vi "PJ1_GG - Copy1.vi"() -> ()   [LabVIEW 2024]
uses:
  contol_vr 23/Control 9.ctl
  <vilib>/Instr/_visa.llb/VISA Configure Serial Port (Instr).vi
  <vilib>/express/express analysis/Spectral/Block/exnSpectralBlock spectral measurements PSD poly.vi
  <vilib>/express/express analysis/Spectral/Block/exnSpectralBlock spectral measurements PSD DDT.vi
  <vilib>/express/express analysis/Spectral/XNode/ExpressSpectralMeasurementsBlockNode.xnode
panel:
  out "Array":dbl[](array[numeric])
  out "appended array 2":dbl[](array[numeric])
  out "element":dbl
  out "data out":string
  in  "Sample":i32
  in  "Rate":dbl
  in  "Upper Cut-Off":dbl=40.0
  out "PSD":dynamicdata(graph)
  out "PSD MAX":dbl
  out "Index ที่มากที่สุด":i32
  out "max value":dbl
  out "B 18+1":dbl
  out "N 18+1":dbl
  in  "Aj 18+1":dbl
  out "B 18+1":dbl
  out "PSD 18+1":dbl
  out "B 18":dbl
  out "N 18":dbl
  in  "Aj 18":dbl
  out "B 18":dbl
  out "PSD 18":dbl
  out "B 18-1":dbl
  out "N 18-1":dbl
  in  "Aj 18-1":dbl
  out "B 18-1":dbl
  out "PSD 18-1":dbl
  out "9 Hz":dbl[](array[numeric])
  out "Max Index 9":i32
  out "PSD max 9":dbl
  out "PSD 9-1":dbl
  out "B 9-1":dbl
  in  "Aj 9-1":dbl
  out "N 9-1":dbl
  out "B 9-1":dbl
  out "PSD 9":dbl
  out "B 9":dbl
  in  "Aj 9":dbl
  out "N 9":dbl
  out "B 9":dbl
  out "PSD 9+1":dbl
  out "B 9+1":dbl
  in  "Aj 9+1":dbl
  out "N 9+1":dbl
  out "B 9+1":dbl
  out "8 Hz":dbl[](array[numeric])
  out "Max Index 8":i32
  out "PSD max 8":dbl
  out "B 16+1":dbl
  out "N 16+1":dbl
  in  "Aj  16+1":dbl
  out "B 16+1":dbl
  out "PSD  16+1":dbl
  out "B 16":dbl
  out "N  16":dbl
  in  "Aj  16":dbl
  out "B 16":dbl
  out "PSD  16":dbl
  out "B 16-1":dbl
  out "N  16-1":dbl
  in  "Aj   16-1":dbl
  out "B   16-1":dbl
  out "PSD 16-1":dbl
  out "B 8+1":dbl
  out "N 8+1":dbl
  in  "Aj  8+1":dbl
  out "B  8+1":dbl
  out "PSD 8+1":dbl
  out "B 8":dbl
  out "N  8":dbl
  in  "Aj  8":dbl
  out "B  8":dbl
  out "PSD 8":dbl
  out "B 8-1":dbl
  out "N  8-1":dbl
  in  "Aj  8-1":dbl
  out "B  8-1":dbl
  out "PSD 8-1":dbl
  out "PSD 14+1":dbl
  out "B 14+1":dbl
  in  "Aj 14+1":dbl
  out "N 14+1":dbl
  out "B 14+1":dbl
  out "PSD 14":dbl
  out "B 14":dbl
  in  "Aj 14":dbl
  out "N 14":dbl
  out "B 14":dbl
  out "PSD 14-1":dbl
  out "B 14-1":dbl
  in  "Aj 14-1":dbl
  out "N 14-1":dbl
  out "B 14-1":dbl
  out "PSD7+1":dbl
  out "B7+1":dbl
  in  "Aj7+1":dbl
  out "N7+1":dbl
  out "B7+1":dbl
  out "PSD 7":dbl
  out "B 7":dbl
  in  "Aj 7":dbl
  out "N7":dbl
  out "B7":dbl
  out "7 Hz":dbl[](array[numeric])
  out "Max Index 7":i32
  out "PSD max 7":dbl
  out "PSD 7-1":dbl
  out "B 7-1":dbl
  in  "Aj 7-1":dbl
  out "N7-1":dbl
  out "B7-1":dbl
  out "B12-1":dbl
  out "N12-1":dbl
  in  "Aj 12-1":dbl
  out "B 12-1":dbl
  out "PSD 12-1":dbl
  out "B12":dbl
  out "N12":dbl
  in  "Aj 12":dbl
  out "B12":dbl
  out "PSD 12":dbl
  out "B12+1":dbl
  out "N12+1":dbl
  in  "Aj 12+1":dbl
  out "B 12+1":dbl
  out "PSD 12+1":dbl
  out "B6+1":dbl
  out "N6+1":dbl
  in  "Aj 6+1":dbl
  out "B 6+1":dbl
  out "PSD 6+1":dbl
  out "B6":dbl
  out "N6":dbl
  in  "Aj 6":dbl
  out "B6":dbl
  out "PSD 6":dbl
  out "PSD 6-1":dbl
  out "6 Hz":dbl[](array[numeric])
  out "Max Index 6":i32
  out "PSD max 6":dbl
  out "B 6-1":dbl
  in  "Aj 6-1":dbl
  out "N6-1":dbl
  out "B6-1":dbl
  in  "Baseline":bool
  out "appended array":dbl[][](array[numeric])
  out "Filtered Signal":dynamicdata(graph)
  in  "Lower Cut-Off":dbl=1.0
  out "?":bool
  out "?":bool
  out "?":bool
  out "?":bool
  out "?":bool
  out "?":bool
  out "?":bool
  out "?":bool
  out "?":bool
  out "?":bool
  out "?":bool=TRUE
  out "?":bool=TRUE
  out "?":bool=TRUE
  out "?":bool=TRUE
  out "?":bool=TRUE
  out "?":bool=TRUE
  out "?":bool=TRUE
  out "?":bool=TRUE
  out "?":bool=TRUE
  out "?":bool=TRUE
  out "?":bool
  out "?":bool
  out "?":bool
  out "?":bool
  out "?":bool
  out "?":bool
  out "?":bool
  out "?":bool
  out "?":bool
  out "?":bool
  out "?":bool=TRUE
  out "?":bool=TRUE
  out "?":bool=TRUE
  out "?":bool=TRUE
  out "?":bool=TRUE
  out "?":bool=TRUE
  out "?":bool=TRUE
  out "?":bool=TRUE
  out "?":bool=TRUE
  out "?":bool=TRUE
  out "?":bool
  out "?":bool
  out "?":bool
  out "?":bool
  out "?":bool
  out "?":bool
  out "?":bool
  out "?":bool
  out "?":bool
  out "?":bool
  out "?":bool=TRUE
  out "?":bool=TRUE
  out "?":bool=TRUE
  out "?":bool=TRUE
  out "?":bool=TRUE
  out "?":bool=TRUE
  out "?":bool=TRUE
  out "?":bool=TRUE
  out "?":bool=TRUE
  out "?":bool=TRUE
  out "?":bool
  out "?":bool
  out "?":bool
  out "?":bool
  out "?":bool
  out "?":bool
  out "?":bool
  out "?":bool
  out "?":bool
  out "?":bool
  out "?":bool=TRUE
  out "?":bool=TRUE
  out "?":bool=TRUE
  out "?":bool=TRUE
  out "?":bool=TRUE
  out "?":bool=TRUE
  out "?":bool=TRUE
  out "?":bool=TRUE
  out "?":bool=TRUE
  out "?":bool=TRUE
  out "9 HZ":bool
  out "8 HZ":bool
  out "6 HZ":bool
  out "7 HZ":bool
  in  "Tab Control":enum32{"TAB 1", "TAB 2", "TAB 3", "TAB 4"}(tab)
  out "555":bool
  in  "MENU 4":bool
  in  "MENU 3":bool
  in  "MENU 2":bool
  in  "MENU":bool
  in  "start":bool
  in  "Text3":bool
  in  "Text2":bool
  in  "Backpage 2":T1
  out "String":string
  in  "Text1":bool
  in  "send":bool
  in  "Back":bool
  in  "1 3":bool
  in  "1 2":bool
  in  "1":bool
  out "String 2":string
  in  "SOS CALLING":bool
  in  "Blank Button 14":bool
  in  "LED":bool
  in  "Blank Button 12":bool
  in  "Back 4":bool
  in  "VISA resource name":refnum<visa-resource-name>
  # "Tel."
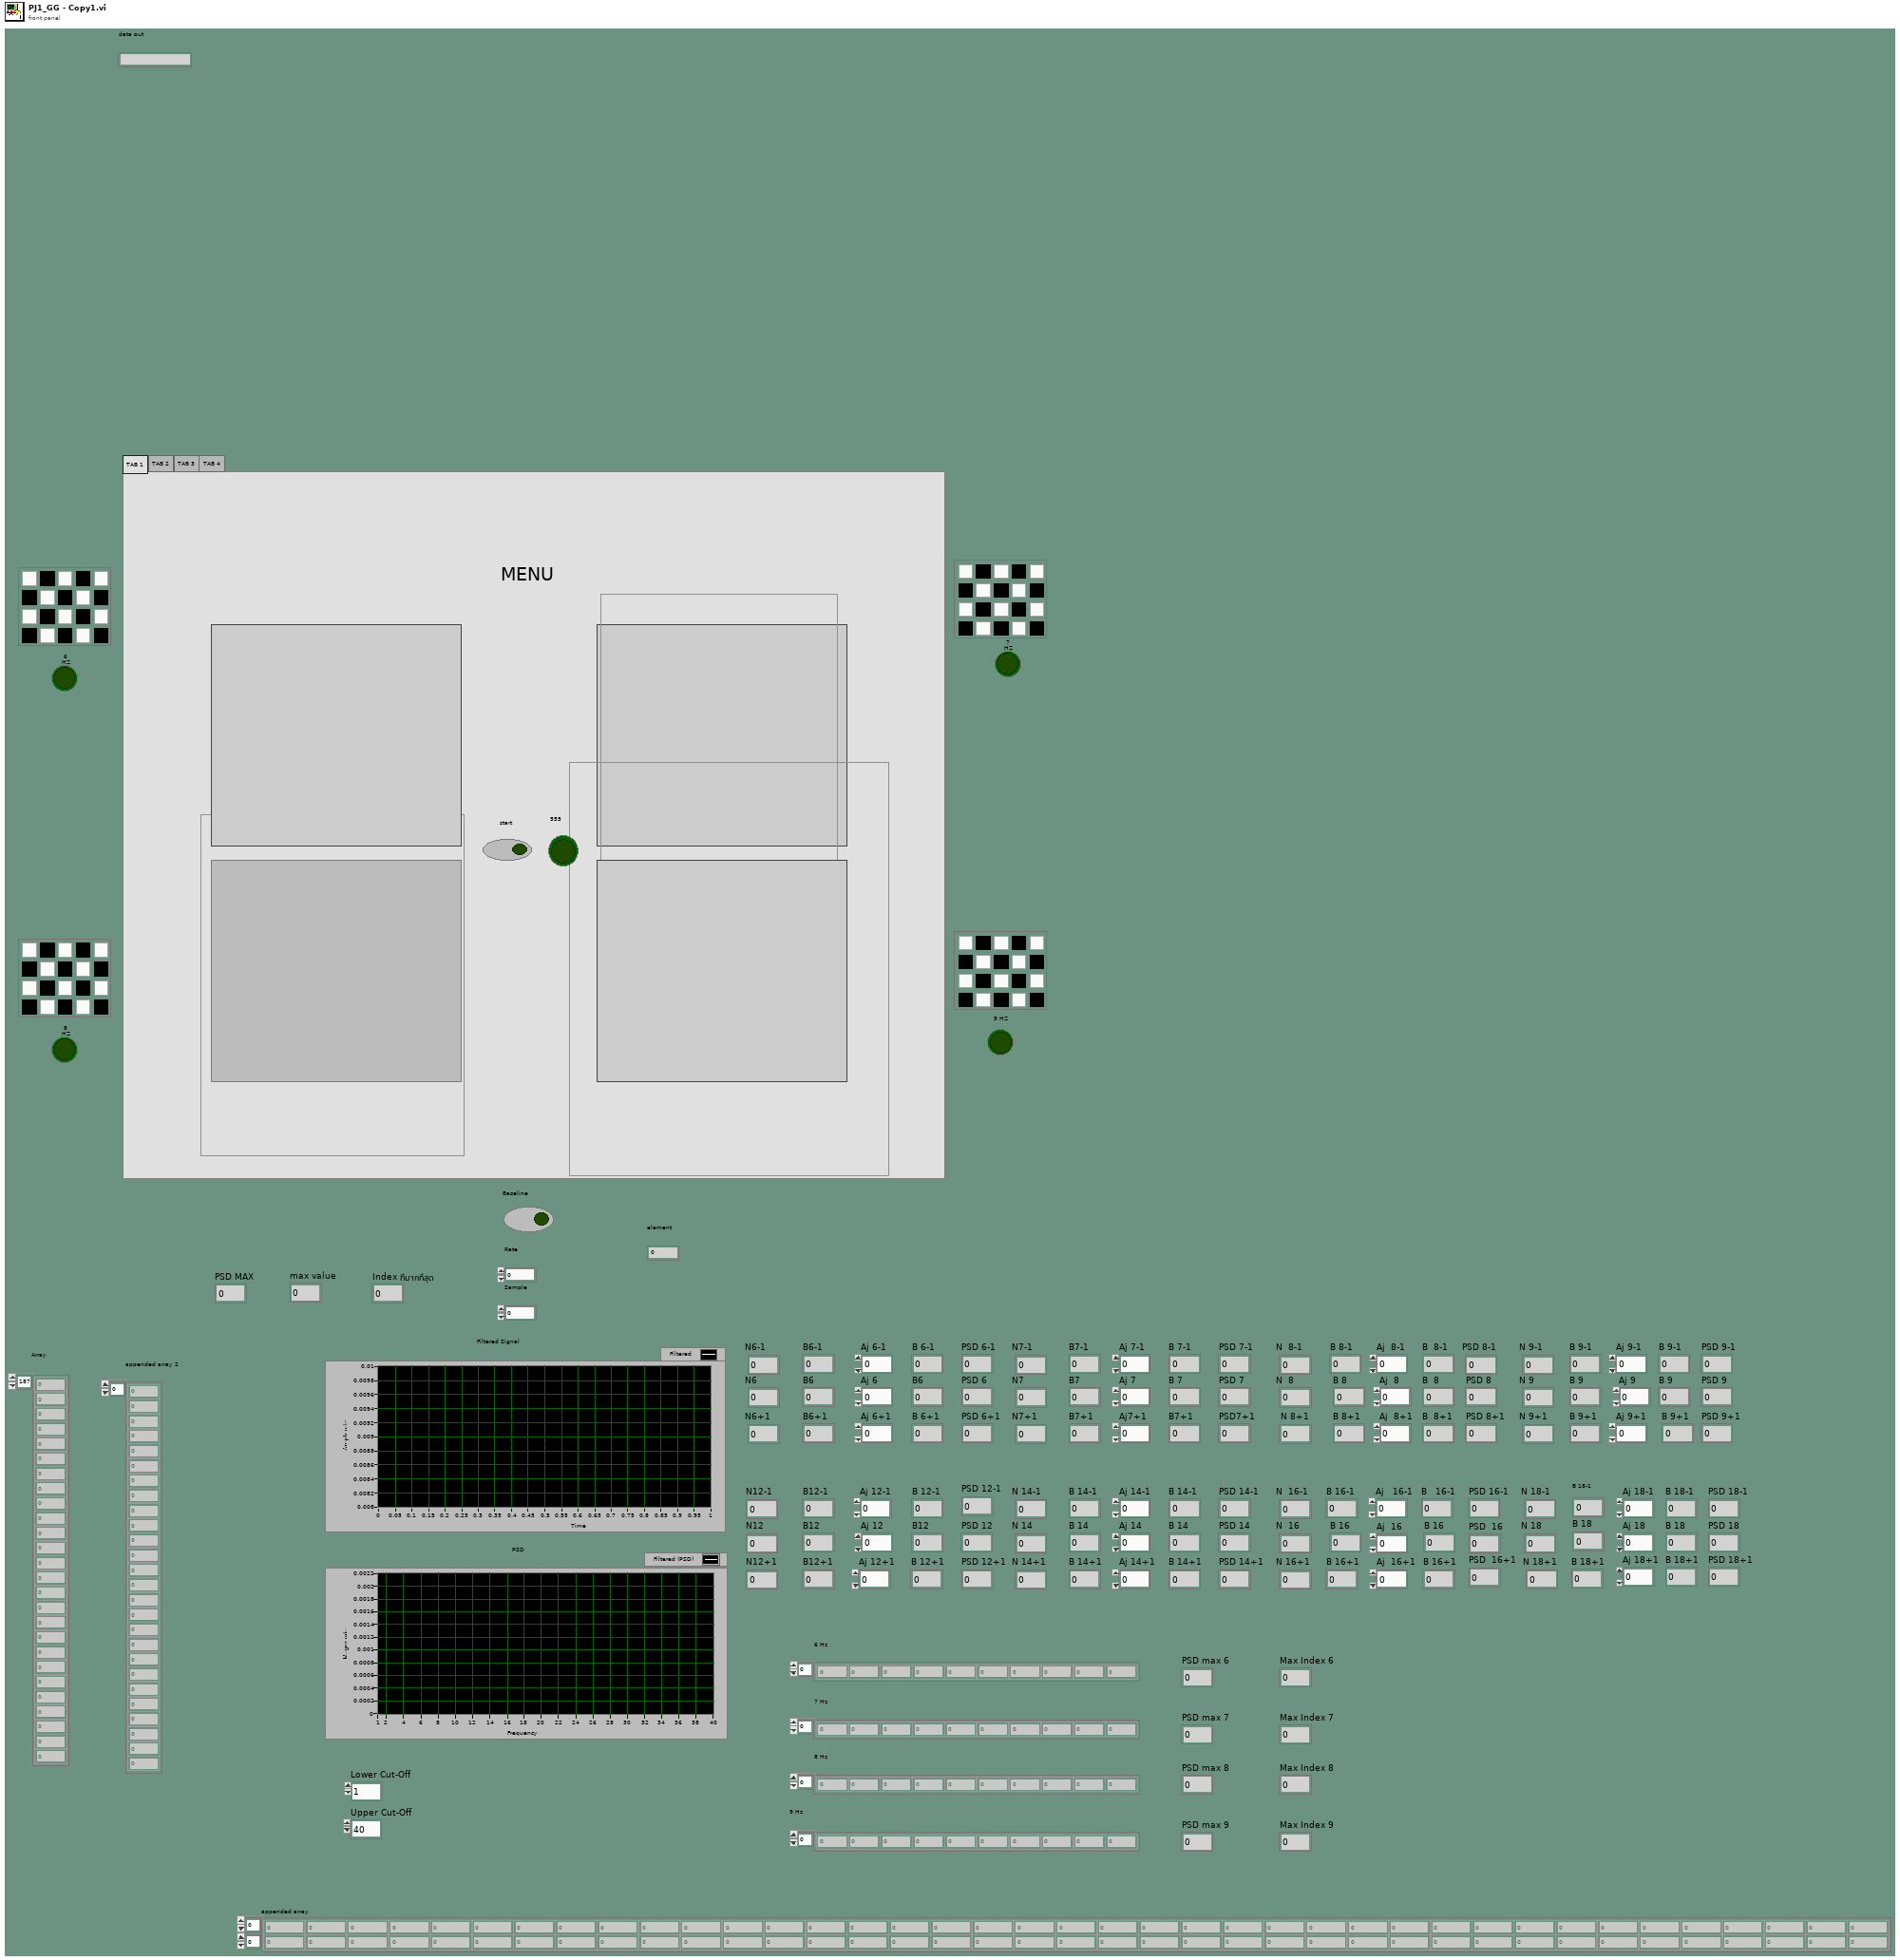
[diagram p1: front panel]
types:
  T1 = typedef "Control 9.ctl" = bool
  T2 = cluster{"averaging mode":u16, "weighting mode":u16, "number of averages":u32}
  T3 = cluster{"dB On (F)":bool, "unwrap phase (F)":bool, "convert to degree (F)":bool}
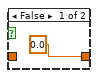
[diagram p3: hidden frame]
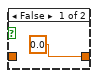
[diagram p5: hidden frame]
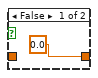
[diagram p7: hidden frame]
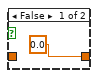
[diagram p9: hidden frame]
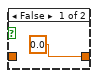
[diagram p11: hidden frame]
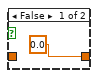
[diagram p13: hidden frame]
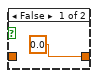
[diagram p15: hidden frame]
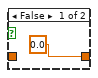
[diagram p17: hidden frame]
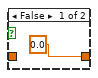
[diagram p19: hidden frame]
diagram:
  n1 = while {
    tunnel: [w15] -> _
    tunnel: [w16] -> _
    stop <- FALSE stop-if-true
    n2 = Obtain Queue(name (unnamed)="buffer", element data type=0.0) -> (queue out=w10:refnum<queue>, error out=w9:errorcluster)  [unwired: 3 in, 1 out]
    n3 = Obtain Queue(name (unnamed)="ganglion", element data type=0.0) -> (queue out=w16:refnum<queue>, error out=w15:errorcluster)  [unwired: 3 in, 1 out]
    n4 = while {
      tunnel: w16 -> [w535]
      tunnel: w15 -> [w534]
      shift-right: [w524] -> _
      shift-left: _ -> [_]
      tunnel: w10 -> [w531]
      tunnel: w9 -> [w530]
      tunnel: [w529] -> w12
      tunnel: [w528] -> w11
      stop <- FALSE stop-if-true
      # "เงื่อนไข while"
      n5 = for {
        N: 200 -> [_]
        shift-right: [w537] -> w524
        shift-left: dbl[] [] -> [w539]
        tunnel: [w544] -> _
        tunnel: w534 -> [w545]
        tunnel: [w541] -> _
        tunnel: [w540] -> _
        tunnel: w535 -> [w544]
        # "เคลีย 800 ก่อน"
        # "ตัด 1 วิเเรกออก"
        n6 = Dequeue Element(queue=w544, error in (no error)=w545) -> (queue out=w540:refnum<queue>, element=w538:dbl, error out=w541:errorcluster)  [unwired: 1 in, 1 out]
        n7 = Build Array (concatenate) "Build Array"(w538, w539) -> (w536:dbl[])
        "appended array 2" <- w536
        n8 = Delete From Array "Delete From Array"(array=w536, length=0, index=199 ("index (row)")) -> (array with subset deleted=w537:dbl[])  [unwired: 1 out]
      }
      "Array" <- w524
      n9 = Index Array(array=w524, index=0) -> (element=w525:dbl)
      "element" <- w525
      n10 = Enqueue Element(queue=w531, element=w525, error in (no error)=w530) -> (queue out=w529:refnum<queue>, error out=w528:errorcluster)  [unwired: 1 in, 1 out]
    }
    n11 = String To IP(1:"127.0.0.1") -> (0:w21:u32)
    n12 = UDP Open(7:w21, 11:u16 5005 ("port")) -> (port=w23:refnum<k16>, 0:w22:errorcluster)  [unwired: 3 in, 1 out]
    n13 = while {
      tunnel: w22 -> [w563]
      tunnel: w23 -> [w561]
      tunnel: [w560] -> w24
      tunnel: [w559] -> w25
      tunnel: [w553] -> w26
      tunnel: w15 -> [w555]
      tunnel: [w554] -> w27
      tunnel: w16 -> [w556]
      stop <- FALSE stop-if-true
      n14 = UDP Read(connection ID=w561, timeout ms (25000)=500, 8:w563) -> (data out=w552:string, error out=w560:errorcluster, 3:w559:refnum<k16>)  [unwired: 1 in, 2 out]
      "data out" <- w552
      n15 = Spreadsheet String To Array(delimiter (Tab)=",", format string="%f", spreadsheet string=w552, array type (2D Dbl)=0.0) -> (array=w550:dbl[][])
      n16 = Index Array(array=w550, index (row)=0, index (col)=0 ("disabled index (col)")) -> (element=w549:dbl)
      n17 = Enqueue Element(queue=w556, element=w549, error in (no error)=w555) -> (queue out=w553:refnum<queue>, error out=w554:errorcluster)  [unwired: 1 in, 1 out]
    }
    n18 = UDP Close(connection ID=w25, 8:w24) -> ()  [unwired: 2 out]
    n19 = Release Queue(queue=w26, error in (no error)=w27) -> ()  [unwired: 1 in, 3 out]
    n20 = Release Queue(queue=w12, error in (no error)=w11) -> ()  [unwired: 1 in, 3 out]
    n21 = while {
      tunnel: w10 -> [w32]
      tunnel: w9 -> [w31]
      stop <- FALSE stop-if-true
      n22 = Dequeue Element(queue=w32, error in (no error)=w31) -> (element=w30:dbl)  [unwired: 1 in, 3 out]
      n23 = Build Array(w30) -> (w29:dbl[])
      n24 = Bundle By Name("dt"=0.005, "Y"=w29) -> (w34:waveform(dbl))  [unwired: 1 in]
      n25 = Divide(x="Rate", y="Sample") -> (x/y=w127:dbl)
      n26 = call "Filter"("Lower Cut-Off"="Lower Cut-Off", "Upper Cut-Off"="Upper Cut-Off", "Signal"=w34) -> ("Filtered Signal"=w36:dynamicdata)  [unwired: 7 in, 1 out]
      "Filtered Signal" <- w36
      n27 = Divide(x=8.0, y=w127) -> (x/y=w227:dbl)
      n28 = Divide(x=16.0, y=w127) -> (x/y=w179:dbl)
      n29 = Divide(x=14.0, y=w127) -> (x/y=w252:dbl)
      n30 = Divide(x=18.0, y=w127) -> (x/y=w102:dbl)
      n31 = xnode "Spectral Measurements"("Signals"=w36) -> ("PSD"=w37:dynamicdata)  [unwired: 1 in, 1 out]
      "PSD" <- w37
      n32 = Divide(x=9.0, y=w127) -> (x/y=w145:dbl)
      n33 = Divide(x=7.0, y=w127) -> (x/y=w269:dbl)
      n34 = Divide(x=12.0, y=w127) -> (x/y=w338:dbl)
      n35 = Divide(x=6.0, y=w127) -> (x/y=w387:dbl)
      n36 = Decrement(x=w145) -> (x-1=w176:dbl)
      n37 = Increment(x=w145) -> (x+1=w144:dbl)
      n38 = call "Convert from Dynamic Data"("Dynamic Data Type"=w37) -> ("Array"=w415:dbl[])  [unwired: 3 in]
      n39 = Increment(x=w102) -> (x+1=w91:dbl)
      n40 = Decrement(x=w102) -> (x-1=w116:dbl)
      n41 = Decrement(x=w252) -> (x-1=w281:dbl)
      n42 = Increment(x=w227) -> (x+1=w217:dbl)
      n43 = Decrement(x=w179) -> (x-1=w202:dbl)
      n44 = Decrement(x=w387) -> (x-1=w400:dbl)
      n45 = Decrement(x=w269) -> (x-1=w310:dbl)
      "PSD 7-1" <- w310
      n46 = Increment(x=w269) -> (x+1=w295:dbl)
      n47 = Decrement(x=w227) -> (x-1=w240:dbl)
      n48 = Increment(x=w179) -> (x+1=w178:dbl)
      n49 = Increment(x=w387) -> (x+1=w376:dbl)
      n50 = Increment(x=w252) -> (x+1=w258:dbl)
      n51 = Decrement(x=w338) -> (x-1=w343:dbl)
      n52 = Increment(x=w338) -> (x+1=w337:dbl)
      n53 = Build Array "Build Array"(w415) -> (w92:dbl[][])
      "appended array" <- w92
      n54 = Index Array(array=w92, index (row)=0, index (col)=w202) -> (element=w213:dbl)
      "PSD 16-1" <- w213
      n55 = Index Array(array=w92, index (row)=0 ("disabled index (row)"), index (col)=w178) -> (element=w190:dbl)
      "PSD  16+1" <- w190
      n56 = Index Array(array=w92, index (row)=0 ("disabled index (row)"), index (col)=w179) -> (element=w192:dbl)
      "PSD  16" <- w192
      n57 = Index Array(array=w92, index (row)=0, index (col)=w258) -> (element=w259:dbl)
      "PSD 14+1" <- w259
      n58 = Index Array(array=w92, index (row)=0 ("disabled index (row)"), index (col)=w116) -> (element=w114:dbl)
      "PSD 18-1" <- w114
      n59 = Index Array(array=w92, index (row)=0, index (col)=w217) -> (element=w215:dbl)
      "PSD 8+1" <- w215
      n60 = Index Array(array=w92, index (row)=0 ("disabled index (row)"), index (col)=w91) -> (element=w88:dbl)
      "PSD 18+1" <- w88
      n61 = Index Array(array=w92, index (row)=0, index (col)=w144) -> (element=w133:dbl)
      "PSD 9-1" <- w133
      n62 = Index Array(array=w92, index (row)=0, index (col)=w227) -> (element=w238:dbl)
      "PSD 8" <- w238
      n63 = Index Array(array=w92, index (row)=0 ("disabled index (row)"), index (col)=w102) -> (element=w103:dbl)
      "PSD 18" <- w103
      n64 = Index Array(array=w92, index (row)=0, index (col)=w240) -> (element=w239:dbl)
      "PSD 8-1" <- w239
      n65 = Index Array(array=w92, index (row)=0, index (col)=w145) -> (element=w146:dbl)
      "PSD 9" <- w146
      n66 = Index Array(array=w92, index (row)=0, index (col)=w176) -> (element=w157:dbl)
      "PSD 9+1" <- w157
      n67 = Index Array(array=w92, index (row)=0, index (col)=w281) -> (element=w283:dbl)
      "PSD 14-1" <- w283
      n68 = Index Array(array=w92, index (row)=0, index (col)=w252) -> (element=w270:dbl)
      "PSD 14" <- w270
      n69 = Index Array(array=w92, index (row)=0, index (col)=w310) -> ()  [unwired: 1 out]
      n70 = Index Array(array=w92, index (row)=0 ("disabled index (row)"), index (col)=w269) -> (element=w307:dbl)
      "PSD 7" <- w307
      n71 = Index Array(array=w92, index (row)=0, index (col)=w295) -> (element=w296:dbl)
      "PSD7+1" <- w296
      n72 = Index Array(array=w92, index (row)=0 ("disabled index (row)"), index (col)=w376) -> (element=w374:dbl)
      "PSD 6+1" <- w374
      n73 = Index Array(array=w92, index (row)=0, index (col)=w343) -> (element=w342:dbl)
      "PSD 12-1" <- w342
      n74 = Index Array(array=w92, index (row)=0 ("disabled index (row)"), index (col)=w338) -> (element=w339:dbl)
      "PSD 12" <- w339
      n75 = Index Array(array=w92, index (row)=0 ("disabled index (row)"), index (col)=w337) -> (element=w335:dbl)
      "PSD 12+1" <- w335
      n76 = Index Array(array=w92, index (row)=0, index (col)=w387) -> (element=w388:dbl)
      "PSD 6" <- w388
      n77 = Index Array(array=w92, index (row)=0, index (col)=w400) -> (element=w407:dbl)
      "PSD 6-1" <- w407
      n78 = feedback #1() -> (w42:dbl)  [unwired: 1 in]
      "B 18" <- w42
      n79 = case shown="False" "Baseline" {
        tunnel: w103 -> [_ w426]
        tunnel: [w425 w426] -> w105
        tunnel: w42 -> [w425 _]
        frame False {
        }
        frame True {
        }
      }
      n80 = feedback-in #1(w105) -> ()
      n81 = feedback #2() -> (w43:dbl)  [unwired: 1 in]
      "B 18-1" <- w43
      n82 = case shown="False" "Baseline" {
        tunnel: w114 -> [_ w430]
        tunnel: [w429 w430] -> w125
        tunnel: w43 -> [w429 _]
        frame False {
        }
        frame True {
        }
      }
      n83 = feedback-in #2(w125) -> ()
      n84 = feedback #3() -> (w41:dbl)  [unwired: 1 in]
      "B 18+1" <- w41
      n85 = case shown="False" "Baseline" {
        tunnel: w88 -> [_ w422]
        tunnel: [w421 w422] -> w101
        tunnel: w41 -> [w421 _]
        frame False {
        }
        frame True {
        }
      }
      n86 = feedback-in #3(w101) -> ()
      n87 = feedback #4() -> (w49:dbl)  [unwired: 1 in]
      "B 16-1" <- w49
      n88 = case shown="True" "Baseline" {
        tunnel: w213 -> [_ w454]
        tunnel: [w453 w454] -> w203
        tunnel: w49 -> [w453 _]
        frame False {
        }
        frame True {
        }
      }
      n89 = feedback-in #4(w203) -> ()
      n90 = feedback #5() -> (w47:dbl)  [unwired: 1 in]
      "B 16+1" <- w47
      n91 = case shown="False" "Baseline" {
        tunnel: w190 -> [_ w446]
        tunnel: [w445 w446] -> w181
        tunnel: w47 -> [w445 _]
        frame False {
        }
        frame True {
        }
      }
      n92 = feedback-in #5(w181) -> ()
      n93 = feedback #6() -> (w48:dbl)  [unwired: 1 in]
      "B 16" <- w48
      n94 = case shown="False" "Baseline" {
        tunnel: w192 -> [_ w450]
        tunnel: [w449 w450] -> w201
        tunnel: w48 -> [w449 _]
        frame False {
        }
        frame True {
        }
      }
      n95 = feedback-in #6(w201) -> ()
      n96 = feedback #7() -> (w50:dbl)  [unwired: 1 in]
      "B 8+1" <- w50
      n97 = case shown="True" "Baseline" {
        tunnel: w215 -> [_ w458]
        tunnel: [w457 w458] -> w226
        tunnel: w50 -> [w457 _]
        frame False {
        }
        frame True {
        }
      }
      n98 = feedback-in #7(w226) -> ()
      n99 = feedback #8() -> (w53:dbl)  [unwired: 1 in]
      "B 14+1" <- w53
      n100 = case shown="True" "Baseline" {
        tunnel: w259 -> [_ w470]
        tunnel: [w469 w470] -> w260
        tunnel: w53 -> [w469 _]
        frame False {
        }
        frame True {
        }
      }
      n101 = feedback-in #8(w260) -> ()
      n102 = feedback #9() -> (w51:dbl)  [unwired: 1 in]
      "B 8" <- w51
      n103 = case shown="True" "Baseline" {
        tunnel: w238 -> [_ w462]
        tunnel: [w461 w462] -> w229
        tunnel: w51 -> [w461 _]
        frame False {
        }
        frame True {
        }
      }
      n104 = feedback-in #9(w229) -> ()
      n105 = feedback #10() -> (w45:dbl)  [unwired: 1 in]
      "B 9" <- w45
      n106 = case shown="False" "Baseline" {
        tunnel: w146 -> [_ w438]
        tunnel: [w437 w438] -> w147
        tunnel: w45 -> [w437 _]
        frame False {
        }
        frame True {
        }
      }
      n107 = feedback-in #10(w147) -> ()
      n108 = feedback #11() -> (w52:dbl)  [unwired: 1 in]
      "B 8-1" <- w52
      n109 = case shown="True" "Baseline" {
        tunnel: w239 -> [_ w466]
        tunnel: [w465 w466] -> w250
        tunnel: w52 -> [w465 _]
        frame False {
        }
        frame True {
        }
      }
      n110 = feedback-in #11(w250) -> ()
      n111 = feedback #12() -> (w46:dbl)  [unwired: 1 in]
      "B 9+1" <- w46
      n112 = case shown="False" "Baseline" {
        tunnel: w157 -> [_ w442]
        tunnel: [w441 w442] -> w158
        tunnel: w46 -> [w441 _]
        frame False {
        }
        frame True {
        }
      }
      n113 = feedback-in #12(w158) -> ()
      n114 = feedback #13() -> (w61:dbl)  [unwired: 1 in]
      "B12-1" <- w61
      n115 = case shown="True" "Baseline" {
        tunnel: w342 -> [_ w502]
        tunnel: [w501 w502] -> w354
        tunnel: w61 -> [w501 _]
        frame False {
        }
        frame True {
        }
      }
      n116 = feedback-in #13(w354) -> ()
      n117 = feedback #14() -> (w55:dbl)  [unwired: 1 in]
      "B 14-1" <- w55
      n118 = case shown="True" "Baseline" {
        tunnel: w283 -> [_ w478]
        tunnel: [w477 w478] -> w284
        tunnel: w55 -> [w477 _]
        frame False {
        }
        frame True {
        }
      }
      n119 = feedback-in #14(w284) -> ()
      n120 = feedback #15() -> (w44:dbl)  [unwired: 1 in]
      "B 9-1" <- w44
      n121 = case shown="False" "Baseline" {
        tunnel: w133 -> [_ w434]
        tunnel: [w433 w434] -> w134
        tunnel: w44 -> [w433 _]
        frame False {
        }
        frame True {
        }
      }
      n122 = feedback-in #15(w134) -> ()
      n123 = feedback #16() -> (w62:dbl)  [unwired: 1 in]
      "B6+1" <- w62
      n124 = case shown="True" "Baseline" {
        tunnel: w374 -> [_ w506]
        tunnel: [w505 w506] -> w377
        tunnel: w62 -> [w505 _]
        frame False {
        }
        frame True {
        }
      }
      n125 = feedback-in #16(w377) -> ()
      n126 = feedback #17() -> (w63:dbl)  [unwired: 1 in]
      "B6" <- w63
      n127 = case shown="True" "Baseline" {
        tunnel: w388 -> [_ w510]
        tunnel: [w509 w510] -> w398
        tunnel: w63 -> [w509 _]
        frame False {
        }
        frame True {
        }
      }
      n128 = feedback-in #17(w398) -> ()
      n129 = feedback #18() -> (w64:dbl)  [unwired: 1 in]
      "B6-1" <- w64
      n130 = case shown="True" "Baseline" {
        tunnel: w407 -> [_ w514]
        tunnel: [w513 w514] -> w399
        tunnel: w64 -> [w513 _]
        frame False {
        }
        frame True {
        }
      }
      n131 = feedback-in #18(w399) -> ()
      n132 = feedback #19() -> (w54:dbl)  [unwired: 1 in]
      "B 14" <- w54
      n133 = case shown="True" "Baseline" {
        tunnel: w270 -> [_ w474]
        tunnel: [w473 w474] -> w272
        tunnel: w54 -> [w473 _]
        frame False {
        }
        frame True {
        }
      }
      n134 = feedback-in #19(w272) -> ()
      n135 = feedback #20() -> (w59:dbl)  [unwired: 1 in]
      "B12+1" <- w59
      n136 = case shown="True" "Baseline" {
        tunnel: w335 -> [_ w494]
        tunnel: [w493 w494] -> w372
        tunnel: w59 -> [w493 _]
        frame False {
        }
        frame True {
        }
      }
      n137 = feedback-in #20(w372) -> ()
      n138 = Add(x=w42, y="Aj 18") -> (x+y=w109:dbl)
      "B 18" <- w109
      n139 = Add(x=w43, y="Aj 18-1") -> (x+y=w121:dbl)
      "B 18-1" <- w121
      n140 = Add(x=w41, y="Aj 18+1") -> (x+y=w97:dbl)
      "B 18+1" <- w97
      n141 = feedback #21() -> (w60:dbl)  [unwired: 1 in]
      "B12" <- w60
      n142 = case shown="True" "Baseline" {
        tunnel: w339 -> [_ w498]
        tunnel: [w497 w498] -> w355
        tunnel: w60 -> [w497 _]
        frame False {
        }
        frame True {
        }
      }
      n143 = feedback-in #21(w355) -> ()
      n144 = Add(x=w49, y="Aj   16-1") -> (x+y=w207:dbl)
      "B   16-1" <- w207
      n145 = Add(x=w47, y="Aj  16+1") -> (x+y=w185:dbl)
      "B 16+1" <- w185
      n146 = Add(x=w48, y="Aj  16") -> (x+y=w197:dbl)
      "B 16" <- w197
      n147 = Add(x=w50, y="Aj  8+1") -> (x+y=w222:dbl)
      "B  8+1" <- w222
      n148 = Add(x=w53, y="Aj 14+1") -> (x+y=w264:dbl)
      "B 14+1" <- w264
      n149 = Add(x=w51, y="Aj  8") -> (x+y=w233:dbl)
      "B  8" <- w233
      n150 = Add(x=w45, y="Aj 9") -> (x+y=w151:dbl)
      "B 9" <- w151
      n151 = Add(x=w52, y="Aj  8-1") -> (x+y=w246:dbl)
      "B  8-1" <- w246
      n152 = Add(x=w46, y="Aj 9+1") -> (x+y=w162:dbl)
      "B 9+1" <- w162
      n153 = Add(x=w61, y="Aj 12-1") -> (x+y=w350:dbl)
      "B 12-1" <- w350
      n154 = Add(x=w55, y="Aj 14-1") -> (x+y=w288:dbl)
      "B 14-1" <- w288
      n155 = Add(x=w44, y="Aj 9-1") -> (x+y=w138:dbl)
      "B 9-1" <- w138
      n156 = Multiply(x=w42, y=5.0) -> (x*y=w112:dbl)
      "N 18" <- w112
      n157 = Add(x=w62, y="Aj 6+1") -> (x+y=w381:dbl)
      "B 6+1" <- w381
      n158 = Multiply(x=w43, y=5.0) -> (x*y=w118:dbl)
      "N 18-1" <- w118
      n159 = Multiply(x=w41, y=5.0) -> (x*y=w94:dbl)
      "N 18+1" <- w94
      n160 = feedback #22() -> (w56:dbl)  [unwired: 1 in]
      "B7+1" <- w56
      n161 = case shown="True" "Baseline" {
        tunnel: w296 -> [_ w482]
        tunnel: [w481 w482] -> w298
        tunnel: w56 -> [w481 _]
        frame False {
        }
        frame True {
        }
      }
      n162 = feedback-in #22(w298) -> ()
      n163 = feedback #23() -> (w57:dbl)  [unwired: 1 in]
      "B7" <- w57
      n164 = case shown="True" "Baseline" {
        tunnel: w307 -> [_ w486]
        tunnel: [w485 w486] -> w311
        tunnel: w57 -> [w485 _]
        frame False {
        }
        frame True {
        }
      }
      n165 = feedback-in #23(w311) -> ()
      n166 = Multiply(x=w49, y=5.0) -> (x*y=w210:dbl)
      "N  16-1" <- w210
      n167 = Multiply(x=w47, y=5.0) -> (x*y=w188:dbl)
      "N 16+1" <- w188
      n168 = Multiply(x=w48, y=5.0) -> (x*y=w194:dbl)
      "N  16" <- w194
      n169 = Multiply(x=w50, y=5.0) -> (x*y=w219:dbl)
      "N 8+1" <- w219
      n170 = feedback #24() -> (w58:dbl)  [unwired: 1 in]
      "B7-1" <- w58
      n171 = case shown="False" "Baseline" {
        tunnel: w310 -> [_ w490]
        tunnel: [w489 w490] -> w324
        tunnel: w58 -> [w489 _]
        frame False {
        }
        frame True {
        }
      }
      n172 = feedback-in #24(w324) -> ()
      n173 = Add(x=w63, y="Aj 6") -> (x+y=w394:dbl)
      "B6" <- w394
      n174 = Add(x=w64, y="Aj 6-1") -> (x+y=w408:dbl)
      "B 6-1" <- w408
      n175 = Add(x=w54, y="Aj 14") -> (x+y=w276:dbl)
      "B 14" <- w276
      n176 = Multiply(x=w53, y=5.0) -> (x*y=w267:dbl)
      "N 14+1" <- w267
      n177 = Multiply(x=w51, y=5.0) -> (x*y=w236:dbl)
      "N  8" <- w236
      n178 = Multiply(x=w45, y=5.0) -> (x*y=w154:dbl)
      "N 9" <- w154
      n179 = Multiply(x=w52, y=5.0) -> (x*y=w243:dbl)
      "N  8-1" <- w243
      n180 = Multiply(x=w46, y=5.0) -> (x*y=w165:dbl)
      "N 9+1" <- w165
      n181 = Add(x=w59, y="Aj 12+1") -> (x+y=w368:dbl)
      "B 12+1" <- w368
      n182 = Multiply(x=w61, y=5.0) -> (x*y=w347:dbl)
      "N12-1" <- w347
      n183 = Multiply(x=w55, y=5.0) -> (x*y=w291:dbl)
      "N 14-1" <- w291
      n184 = Add(x=w60, y="Aj 12") -> (x+y=w359:dbl)
      "B12" <- w359
      n185 = Multiply(x=w44, y=5.0) -> (x*y=w141:dbl)
      "N 9-1" <- w141
      n186 = Multiply(x=w62, y=5.0) -> (x*y=w384:dbl)
      "N6+1" <- w384
      n187 = Greater?(x=w103, y=w109) -> (0:w110:bool)
      n188 = Greater?(x=w114, y=w121) -> (0:w120:bool)
      n189 = Greater?(x=w88, y=w97) -> (0:w96:bool)
      n190 = Less?(x=w103, y=w112) -> (x < y?=w111:bool)
      n191 = Less?(x=w114, y=w118) -> (x < y?=w119:bool)
      n192 = Multiply(x=w63, y=5.0) -> (x*y=w391:dbl)
      "N6" <- w391
      n193 = Multiply(x=w64, y=5.0) -> (x*y=w411:dbl)
      "N6-1" <- w411
      n194 = Multiply(x=w54, y=5.0) -> (x*y=w279:dbl)
      "N 14" <- w279
      n195 = Greater?(x=w213, y=w207) -> (0:w208:bool)
      n196 = Less?(x=w88, y=w94) -> (x < y?=w95:bool)
      n197 = Greater?(x=w190, y=w185) -> (0:w186:bool)
      n198 = Greater?(x=w192, y=w197) -> (0:w196:bool)
      n199 = Greater?(x=w215, y=w222) -> (0:w221:bool)
      n200 = Less?(x=w213, y=w210) -> (x < y?=w209:bool)
      n201 = Less?(x=w190, y=w188) -> (x < y?=w187:bool)
      n202 = Multiply(x=w59, y=5.0) -> (x*y=w365:dbl)
      "N12+1" <- w365
      n203 = Less?(x=w192, y=w194) -> (x < y?=w195:bool)
      n204 = Greater?(x=w259, y=w264) -> (0:w265:bool)
      n205 = Less?(x=w215, y=w219) -> (x < y?=w220:bool)
      n206 = Greater?(x=w238, y=w233) -> (0:w234:bool)
      n207 = Greater?(x=w146, y=w151) -> (0:w152:bool)
      n208 = Multiply(x=w60, y=5.0) -> (x*y=w362:dbl)
      "N12" <- w362
      n209 = Add(x=w56, y="Aj7+1") -> (x+y=w302:dbl)
      "B7+1" <- w302
      n210 = Less?(x=w259, y=w267) -> (x < y?=w266:bool)
      n211 = Greater?(x=w239, y=w246) -> (0:w245:bool)
      n212 = Less?(x=w238, y=w236) -> (x < y?=w235:bool)
      n213 = Less?(x=w146, y=w154) -> (x < y?=w153:bool)
      n214 = Greater?(x=w157, y=w162) -> (0:w163:bool)
      n215 = Add(x=w57, y="Aj 7") -> (x+y=w315:dbl)
      "B 7" <- w315
      n216 = Less?(x=w239, y=w243) -> (x < y?=w244:bool)
      n217 = Greater?(x=w342, y=w350) -> (0:w349:bool)
      n218 = Greater?(x=w283, y=w288) -> (0:w289:bool)
      n219 = Less?(x=w157, y=w165) -> (x < y?=w164:bool)
      n220 = Greater?(x=w133, y=w138) -> (0:w139:bool)
      n221 = Add(x=w58, y="Aj 7-1") -> (x+y=w328:dbl)
      "B 7-1" <- w328
      n222 = Greater?(x=w374, y=w381) -> (0:w382:bool)
      n223 = Less?(x=w342, y=w347) -> (x < y?=w348:bool)
      n224 = Less?(x=w283, y=w291) -> (x < y?=w290:bool)
      n225 = Less?(x=w133, y=w141) -> (x < y?=w140:bool)
      n226 = Less?(x=w374, y=w384) -> (x < y?=w383:bool)
      n227 = And(x=w111, y=w110) -> (x .and. y?=w108:bool)
      n228 = Subtract(x=w103, y=w109) -> (x-y=w107:dbl)
      n229 = And(x=w119, y=w120) -> (x .and. y?=w122:bool)
      n230 = Greater?(x=w388, y=w394) -> (0:w393:bool)
      n231 = Subtract(x=w114, y=w121) -> (x-y=w123:dbl)
      n232 = Greater?(x=w407, y=w408) -> (0:w409:bool)
      n233 = Greater?(x=w270, y=w276) -> (0:w277:bool)
      n234 = And(x=w95, y=w96) -> (x .and. y?=w98:bool)
      n235 = Subtract(x=w88, y=w97) -> (x-y=w99:dbl)
      n236 = Less?(x=w388, y=w391) -> (x < y?=w392:bool)
      n237 = Less?(x=w407, y=w411) -> (x < y?=w410:bool)
      n238 = Less?(x=w270, y=w279) -> (x < y?=w278:bool)
      n239 = And(x=w209, y=w208) -> (x .and. y?=w206:bool)
      n240 = Multiply(x=w56, y=5.0) -> (x*y=w305:dbl)
      "N7+1" <- w305
      n241 = Subtract(x=w213, y=w207) -> (x-y=w205:dbl)
      n242 = And(x=w187, y=w186) -> (x .and. y?=w184:bool)
      n243 = Subtract(x=w190, y=w185) -> (x-y=w183:dbl)
      n244 = Greater?(x=w335, y=w368) -> (0:w367:bool)
      n245 = Multiply(x=w57, y=5.0) -> (x*y=w318:dbl)
      "N7" <- w318
      n246 = And(x=w195, y=w196) -> (x .and. y?=w198:bool)
      n247 = And(x=w220, y=w221) -> (x .and. y?=w223:bool)
      n248 = Subtract(x=w192, y=w197) -> (x-y=w199:dbl)
      n249 = Subtract(x=w215, y=w222) -> (x-y=w224:dbl)
      n250 = Greater?(x=w339, y=w359) -> (0:w360:bool)
      n251 = Less?(x=w335, y=w365) -> (x < y?=w366:bool)
      n252 = And(x=w266, y=w265) -> (x .and. y?=w263:bool)
      n253 = Subtract(x=w259, y=w264) -> (x-y=w262:dbl)
      n254 = Multiply(x=w58, y=5.0) -> (x*y=w331:dbl)
      "N7-1" <- w331
      n255 = And(x=w235, y=w234) -> (x .and. y?=w232:bool)
      n256 = Subtract(x=w238, y=w233) -> (x-y=w231:dbl)
      n257 = And(x=w153, y=w152) -> (x .and. y?=w150:bool)
      n258 = Subtract(x=w146, y=w151) -> (x-y=w149:dbl)
      n259 = Less?(x=w339, y=w362) -> (x < y?=w361:bool)
      n260 = And(x=w244, y=w245) -> (x .and. y?=w247:bool)
      n261 = Subtract(x=w239, y=w246) -> (x-y=w248:dbl)
      n262 = And(x=w164, y=w163) -> (x .and. y?=w161:bool)
      n263 = Subtract(x=w157, y=w162) -> (x-y=w160:dbl)
      n264 = And(x=w348, y=w349) -> (x .and. y?=w351:bool)
      n265 = Subtract(x=w342, y=w350) -> (x-y=w352:dbl)
      n266 = And(x=w290, y=w289) -> (x .and. y?=w287:bool)
      n267 = Subtract(x=w283, y=w288) -> (x-y=w286:dbl)
      n268 = And(x=w140, y=w139) -> (x .and. y?=w137:bool)
      n269 = Subtract(x=w133, y=w138) -> (x-y=w136:dbl)
      n270 = Subtract(x=w374, y=w381) -> (x-y=w379:dbl)
      n271 = And(x=w383, y=w382) -> (x .and. y?=w380:bool)
      n272 = And(x=w410, y=w409) -> (x .and. y?=w406:bool)
      n273 = Subtract(x=w388, y=w394) -> (x-y=w396:dbl)
      n274 = And(x=w278, y=w277) -> (x .and. y?=w275:bool)
      n275 = Subtract(x=w407, y=w408) -> (x-y=w405:dbl)
      n276 = Greater?(x=w296, y=w302) -> (0:w303:bool)
      n277 = Subtract(x=w270, y=w276) -> (x-y=w274:dbl)
      n278 = Greater?(x=w307, y=w315) -> (0:w316:bool)
      n279 = And(x=w392, y=w393) -> (x .and. y?=w395:bool)
      n280 = Less?(x=w296, y=w305) -> (x < y?=w304:bool)
      n281 = Less?(x=w307, y=w318) -> (x < y?=w317:bool)
      n282 = Subtract(x=w335, y=w368) -> (x-y=w370:dbl)
      n283 = Greater?(x=w310, y=w328) -> (0:w329:bool)
      n284 = Subtract(x=w339, y=w359) -> (x-y=w357:dbl)
      n285 = And(x=w366, y=w367) -> (x .and. y?=w369:bool)
      n286 = Less?(x=w310, y=w331) -> (x < y?=w330:bool)
      n287 = And(x=w361, y=w360) -> (x .and. y?=w358:bool)
      n288 = And(x=w304, y=w303) -> (x .and. y?=w301:bool)
      n289 = Subtract(x=w296, y=w302) -> (x-y=w300:dbl)
      n290 = And(x=w317, y=w316) -> (x .and. y?=w314:bool)
      n291 = Subtract(x=w307, y=w315) -> (x-y=w313:dbl)
      n292 = And(x=w330, y=w329) -> (x .and. y?=w327:bool)
      n293 = Subtract(x=w310, y=w328) -> (x-y=w326:dbl)
      n294 = case shown="True" w351 {
        tunnel: w352 -> [_ w500]
        tunnel: [0.0 w500] -> w341
        frame False {
        }
        frame True {
        }
      }
      n295 = case shown="True" w380 {
        tunnel: w379 -> [_ w504]
        tunnel: [0.0 w504] -> w373
        frame False {
        }
        frame True {
        }
      }
      n296 = case shown="True" w406 {
        tunnel: w405 -> [_ w512]
        tunnel: [0.0 w512] -> w403
        frame False {
        }
        frame True {
        }
      }
      n297 = case shown="False" w395 {
        tunnel: w396 -> [_ w508]
        tunnel: [0.0 w508] -> w386
        frame False {
        }
        frame True {
        }
      }
      n298 = case shown="True" w369 {
        tunnel: w370 -> [_ w492]
        tunnel: [0.0 w492] -> w333
        frame False {
        }
        frame True {
        }
      }
      n299 = case shown="True" w108 {
        tunnel: w107 -> [_ w424]
        tunnel: [0.0 w424] -> w86
        frame False {
        }
        frame True {
        }
      }
      n300 = case shown="True" w358 {
        tunnel: w357 -> [_ w496]
        tunnel: [0.0 w496] -> w334
        frame False {
        }
        frame True {
        }
      }
      n301 = case shown="True" w122 {
        tunnel: w123 -> [_ w428]
        tunnel: [0.0 w428] -> w87
        frame False {
        }
        frame True {
        }
      }
      n302 = case shown="True" w98 {
        tunnel: w99 -> [_ w420]
        tunnel: [0.0 w420] -> w85
        frame False {
        }
        frame True {
        }
      }
      n303 = case shown="True" w206 {
        tunnel: w205 -> [_ w452]
        tunnel: [0.0 w452] -> w169
        frame False {
        }
        frame True {
        }
      }
      n304 = case shown="True" w184 {
        tunnel: w183 -> [_ w444]
        tunnel: [0.0 w444] -> w167
        frame False {
        }
        frame True {
        }
      }
      n305 = case shown="True" w198 {
        tunnel: w199 -> [_ w448]
        tunnel: [0.0 w448] -> w168
        frame False {
        }
        frame True {
        }
      }
      n306 = case shown="True" w223 {
        tunnel: w224 -> [_ w456]
        tunnel: [0.0 w456] -> w170
        frame False {
        }
        frame True {
        }
      }
      n307 = case shown="True" w263 {
        tunnel: w262 -> [_ w468]
        tunnel: [0.0 w468] -> w254
        frame False {
        }
        frame True {
        }
      }
      n308 = case shown="True" w232 {
        tunnel: w231 -> [_ w460]
        tunnel: [0.0 w460] -> w171
        frame False {
        }
        frame True {
        }
      }
      n309 = case shown="True" w275 {
        tunnel: w274 -> [_ w472]
        tunnel: [0.0 w472] -> w255
        frame False {
        }
        frame True {
        }
      }
      n310 = case shown="True" w150 {
        tunnel: w149 -> [_ w436]
        tunnel: [0.0 w436] -> w129
        frame False {
        }
        frame True {
        }
      }
      n311 = case shown="True" w247 {
        tunnel: w248 -> [_ w464]
        tunnel: [0.0 w464] -> w172
        frame False {
        }
        frame True {
        }
      }
      n312 = case shown="True" w287 {
        tunnel: w286 -> [_ w476]
        tunnel: [0.0 w476] -> w256
        frame False {
        }
        frame True {
        }
      }
      n313 = case shown="True" w301 {
        tunnel: w300 -> [_ w480]
        tunnel: [0.0 w480] -> w293
        frame False {
        }
        frame True {
        }
      }
      n314 = case shown="True" w161 {
        tunnel: w160 -> [_ w440]
        tunnel: [0.0 w440] -> w130
        frame False {
        }
        frame True {
        }
      }
      n315 = case shown="True" w314 {
        tunnel: w313 -> [_ w484]
        tunnel: [0.0 w484] -> w294
        frame False {
        }
        frame True {
        }
      }
      n316 = case shown="True" w137 {
        tunnel: w136 -> [_ w432]
        tunnel: [0.0 w432] -> w128
        frame False {
        }
        frame True {
        }
      }
      n317 = case shown="False" w327 {
        tunnel: w326 -> [_ w488]
        tunnel: [0.0 w488] -> w320
        frame False {
        }
        frame True {
        }
      }
      n318 = Build Array(w320, w294, w293, w256, w255, w254) -> (w321:dbl[])
      "7 Hz" <- w321
      n319 = Build Array(w403, w386, w373, w341, w334, w333) -> (w401:dbl[])
      "6 Hz" <- w401
      n320 = Array Max & Min(array=w321) -> (max value=w84:dbl, max index (indices)=→"Max Index 7":i32)  [unwired: 2 out]
      "PSD max 7" <- w84
      n321 = Array Max & Min(array=w401) -> (max value=w81:dbl, max index (indices)=→"Max Index 6":i32)  [unwired: 2 out]
      "PSD max 6" <- w81
      n322 = Build Array(w172, w171, w170, w169, w168, w167) -> (w173:dbl[])
      "8 Hz" <- w173
      n323 = Build Array(w130, w129, w128, w87, w86, w85) -> (w131:dbl[])
      "9 Hz" <- w131
      n324 = Array Max & Min(array=w173) -> (max value=w83:dbl, max index (indices)=→"Max Index 8":i32)  [unwired: 2 out]
      "PSD max 8" <- w83
      n325 = Array Max & Min(array=w131) -> (max value=w82:dbl, max index (indices)=→"Max Index 9":i32)  [unwired: 2 out]
      "PSD max 9" <- w82
      n326 = Build Array(w81, w84, w83, w82) -> (w80:dbl[])
      n327 = Array Max & Min(array=w80) -> (max value=w78:dbl, max index (indices)=w79:i32)  [unwired: 2 out]
      "max value" <- w78
      "PSD MAX" <- w78
      n328 = Greater?(x=w78, y=0.0 ("x")) -> (0:w76:bool)
      n329 = case shown="False" w76 {
        tunnel: w79 -> [_ w418]
        tunnel: [555 w418] -> w66
        frame False {
        }
        frame True {
        }
      }
      "Index ที่มากที่สุด" <- w66
      n330 = Equal?(x=0, y=w66) -> (x = y?=→"6 HZ":bool)
      n331 = Equal?(x=1, y=w66) -> (x = y?=→"7 HZ":bool)
      n332 = Equal?(x=2, y=w66) -> (x = y?=→"9 HZ":bool)
      n333 = Equal?(x=3, y=w66) -> (x = y?=→"8 HZ":bool)
      n334 = Equal?(x=555, y=w66) -> (x = y?=→"555":bool)
    }
  }
  n335 = while {
    shift-right: [w564] -> _
    shift-left: "" -> [w566]
    stop <- FALSE stop-if-true
    n336 = event shown="[3] \"Back\": Value Change" {
      selector: _ -> [_ _ _ _]
      dyn-events: _ -> [_ _ _ _]
      timeout: _ -> [_ _ _ _]
      tunnel: w566 -> [_ _ _ _]
      tunnel: ["0622436287" "1669" " 0937529340" _] -> w564
      event "1 2": Value Change {
        n337 = event-data() -> ()  [unwired: 1 in, 6 out]
      }
      event "1": Value Change {
        n338 = event-data() -> ()  [unwired: 1 in, 6 out]
      }
      event "1 3": Value Change {
        n339 = event-data() -> ()  [unwired: 1 in, 6 out]
      }
      event "Back": Value Change {
        n340 = event-data() -> ()  [unwired: 1 in, 6 out]
        n341 = local write "Tab Control"(enum32{"TAB 1", "TAB 2", "TAB 3", "TAB 4"}."TAB 1" ("Tab Control")) -> ()
      }
    }
    "String 2" <- w564
  }
  n342 = while {
    stop <- FALSE stop-if-true
    n343 = while {
      tunnel: "start" -> [_]
      stop <- FALSE stop-if-true
      n344 = while {
        stop <- FALSE stop-if-true
        w611 = 83.3333
        # "6 HZ"
        n345 = for {
          N: 2 -> [_]
          tunnel: w611 -> [w615]
          i -> [w617]
          n346 = Wait (ms)(milliseconds to wait=w615) -> ()  [unwired: 1 out]
          n347 = Equal?(x=0, y=w617) -> (x = y?=→"?" →"?" →"?" →"?" →"?" →"?" →"?" →"?" →"?" →"?":bool)
        }
        n348 = for {
          N: 2 -> [_]
          tunnel: w611 -> [w619]
          i -> [w620]
          n349 = Wait (ms)(milliseconds to wait=w619) -> ()  [unwired: 1 out]
          n350 = Equal?(x=1, y=w620) -> (x = y?=→"?" →"?" →"?" →"?" →"?" →"?" →"?" →"?" →"?" →"?":bool)
        }
      }
      n351 = while {
        stop <- FALSE stop-if-true
        w599 = 71.428571
        # "7 HZ"
        n352 = for {
          N: 2 -> [_]
          tunnel: w599 -> [w603]
          i -> [w605]
          n353 = Wait (ms)(milliseconds to wait=w603) -> ()  [unwired: 1 out]
          n354 = Equal?(x=0, y=w605) -> (x = y?=→"?" →"?" →"?" →"?" →"?" →"?" →"?" →"?" →"?" →"?":bool)
        }
        n355 = for {
          N: 2 -> [_]
          tunnel: w599 -> [w607]
          i -> [w608]
          n356 = Wait (ms)(milliseconds to wait=w607) -> ()  [unwired: 1 out]
          n357 = Equal?(x=1, y=w608) -> (x = y?=→"?" →"?" →"?" →"?" →"?" →"?" →"?" →"?" →"?" →"?":bool)
        }
      }
      n358 = while {
        stop <- FALSE stop-if-true
        w587 = 62.5
        # "8 HZ"
        n359 = for {
          N: 2 -> [_]
          tunnel: w587 -> [w591]
          i -> [w593]
          n360 = Wait (ms)(milliseconds to wait=w591) -> ()  [unwired: 1 out]
          n361 = Equal?(x=0, y=w593) -> (x = y?=→"?" →"?" →"?" →"?" →"?" →"?" →"?" →"?" →"?" →"?":bool)
        }
        n362 = for {
          N: 2 -> [_]
          tunnel: w587 -> [w595]
          i -> [w596]
          n363 = Wait (ms)(milliseconds to wait=w595) -> ()  [unwired: 1 out]
          n364 = Equal?(x=1, y=w596) -> (x = y?=→"?" →"?" →"?" →"?" →"?" →"?" →"?" →"?" →"?" →"?":bool)
        }
      }
      n365 = while {
        stop <- FALSE stop-if-true
        w575 = 55.5555
        # "9 HZ"
        n366 = for {
          N: 2 -> [_]
          tunnel: w575 -> [w579]
          i -> [w581]
          n367 = Wait (ms)(milliseconds to wait=w579) -> ()  [unwired: 1 out]
          n368 = Equal?(x=0, y=w581) -> (x = y?=→"?" →"?" →"?" →"?" →"?" →"?" →"?" →"?" →"?" →"?":bool)
        }
        n369 = for {
          N: 2 -> [_]
          tunnel: w575 -> [w583]
          i -> [w584]
          n370 = Wait (ms)(milliseconds to wait=w583) -> ()  [unwired: 1 out]
          n371 = Equal?(x=1, y=w584) -> (x = y?=→"?" →"?" →"?" →"?" →"?" →"?" →"?" →"?" →"?" →"?":bool)
        }
      }
    }
  }
  n372 = while {
    stop <- FALSE stop-if-true
    n373 = event shown="[3] \"MENU 2\": Value Change" {
      selector: _ -> [_ _ _ _ _ _ _]
      dyn-events: _ -> [_ _ _ _ _ _ _]
      timeout: _ -> [_ _ _ _ _ _ _]
      event Timeout {
        n374 = event-data() -> ()  [unwired: 1 in, 3 out]
      }
      event "MENU": Value Change {
        n375 = event-data() -> ()  [unwired: 1 in, 6 out]
        n376 = local write "Tab Control"(enum32{"TAB 1", "TAB 2", "TAB 3", "TAB 4"}."TAB 2" ("Tab Control")) -> ()
      }
      event Value Change {
        n377 = event-data() -> ()  [unwired: 1 in, 6 out]
        n378 = local write "Tab Control"(enum32{"TAB 1", "TAB 2", "TAB 3", "TAB 4"}."TAB 1" ("Tab Control")) -> ()
      }
      event "MENU 2": Value Change {
        n379 = event-data() -> ()  [unwired: 1 in, 6 out]
        n380 = local write "Tab Control"(enum32{"TAB 1", "TAB 2", "TAB 3", "TAB 4"}."TAB 3" ("Tab Control")) -> ()
      }
      event "MENU 3": Value Change {
        n381 = event-data() -> ()  [unwired: 1 in, 6 out]
        n382 = local write "Tab Control"(enum32{"TAB 1", "TAB 2", "TAB 3", "TAB 4"}."TAB 4" ("Tab Control")) -> ()
      }
      event "MENU 4": Value Change {
        n383 = event-data() -> ()  [unwired: 1 in, 6 out]
        n384 = local write "Tab Control"(enum32{"TAB 1", "TAB 2", "TAB 3", "TAB 4"}."TAB 4" ("Tab Control")) -> ()
      }
      event "Back 4": Value Change {
        n385 = event-data() -> ()  [unwired: 1 in, 6 out]
        n386 = local write "Tab Control"(enum32{"TAB 1", "TAB 2", "TAB 3", "TAB 4"}."TAB 1" ("Tab Control")) -> ()
      }
    }
  }
  n387 = while {
    shift-right: [w629] -> _
    shift-left: "" -> [w631]
    stop <- FALSE stop-if-true
    n388 = event shown="[0] \"Text1\": Value Change" {
      selector: _ -> [_ _ _]
      dyn-events: _ -> [_ _ _]
      timeout: _ -> [_ _ _]
      tunnel: w631 -> [_ _ _]
      tunnel: ["ช่วยด้วย ฉันต้องการความช่วยเหลือ !!!" "ฉันต้องการรับประทานอาหาร" "ฉันมีโรคประจำตัว และรู้สึกอาการกำเริบ !!!"] -> w629
      event "Text1": Value Change {
        n389 = event-data() -> ()  [unwired: 1 in, 6 out]
      }
      event "Text2": Value Change {
        n390 = event-data() -> ()  [unwired: 1 in, 6 out]
      }
      event "Text3": Value Change {
        n391 = event-data() -> ()  [unwired: 1 in, 6 out]
      }
    }
    "String" <- w629
  }
  n392 = call-poly "VISA Configure Serial Port"("VISA resource name"="VISA resource name", "baud rate (9600)"=u32 9600) -> ("VISA resource name out"=w7:refnum<visa-resource-name>, "error out"=w5:errorcluster)  [unwired: 12 in]
  n393 = while {
    shift-right: [w643] -> w6
    shift-left: w7 -> [w644]
    shift-right: [w641] -> w4
    shift-left: w5 -> [w642]
    stop <- FALSE stop-if-true
    n394 = Select(t="a", s="LED", f="b") -> (s? t:f=w638:string)
    n395 = VISA Write(VISA resource name=w644, write buffer=w638, error in (no error)=w642) -> (VISA resource name out=w643:refnum<visa-resource-name>, error out=w641:errorcluster)  [unwired: 1 out]
    n396 = Wait (ms)(milliseconds to wait=u32 5) -> ()  [unwired: 1 out]
  }
  n397 = VISA Close(VISA resource name=w6, error in (no error)=w4) -> ()  [unwired: 1 out]
